vi "Сумматор(одноразрядный).vi"(2 "c-1":bool, 3 "b":bool, 4 "a":bool) -> (0 "c":bool, 1 "s":bool)   [LabVIEW 2013]
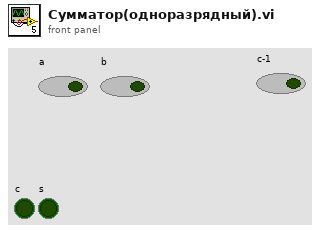
[diagram p1: front panel]
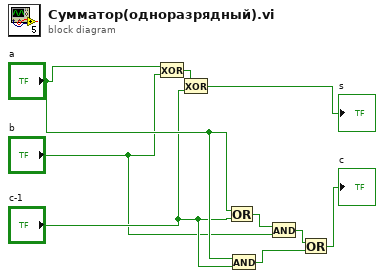
[diagram p0: block diagram]
diagram:
  n1 = Exclusive Or(1:"b", 2:"a") -> (0:w9:bool)
  n2 = Exclusive Or(1:"c-1", 2:w9) -> (0:→"s":bool)
  n3 = Or(x="a", y="c-1") -> (x .or. y?=w5:bool)
  n4 = And(x="a", y="c-1") -> (x .and. y?=w2:bool)
  n5 = And(x=w5, y="b") -> (x .and. y?=w3:bool)
  n6 = Or(x=w3, y=w2) -> (x .or. y?=→"c":bool)
